vi "getPhysicalChannels.vi"(8 "error in (no error)":errorcluster, 11 "DeviceData in":refnum<class "DeviceData.lvclass">) -> (0 "error out":errorcluster, 2 "physicalChannels":string, 3 "DeviceData out":refnum<class "DeviceData.lvclass">)   [LabVIEW 2009, in "DataMappers.lvlib" / "DeviceData.lvclass"]
uses:
  DeviceData.lvclass
  Scripting/ScriptingEvent/ScriptEventList/ScriptEventList.lvclass
  DeviceData.lvclass/DeviceData.ctl
  DatabaseHelpers/Database Objects/device/device.lvclass
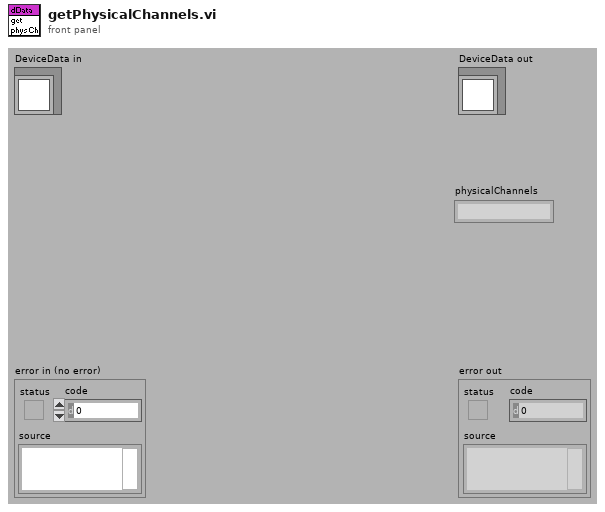
[diagram p1: front panel]
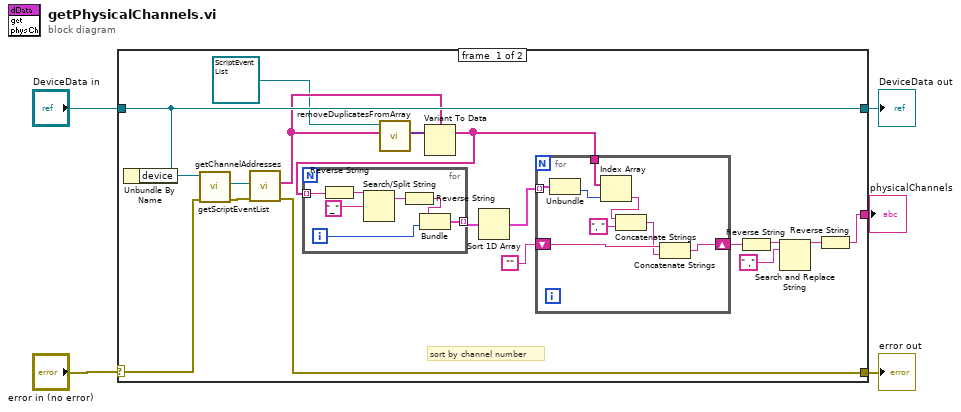
[diagram p0: block diagram]
diagram:
  n1 = case shown="No Error" "error in (no error)" {
    selector: "error in (no error)" -> [w13 w40]
    tunnel: [w12 w40] -> w4
    tunnel: [w23 w39] -> w2
    tunnel: "DeviceData in" -> [w23 w39]
    tunnel: [w14 _] -> w1
    frame #0 {
      # "sort by channel number"
      n2 = Unbundle By Name(w23) -> ("device"=w22:refnum<class "device.lvclass">)
      n3 = call "getScriptEventList.vi"("error in (no error)"=w13, "device.lvclass in"=w22) -> ("error out"=w20:errorcluster, "ScriptEventList"=w21:refnum<class "ScriptEventList.lvclass">)  [unwired: 7 in, 1 out]
      n4 = call "getChannelAddresses.vi"("error in (no error)"=w20, "ScriptEventList in"=w21) -> ("error out"=w12:errorcluster, "ChannelAddresses"=w8:string[])  [unwired: 7 in, 1 out]
      n5 = call "removeDuplicatesFromArray.vi"("Array"=w8, "ScriptEventList in"=refnum<class "ScriptEventList.lvclass"> refnum) -> ("Array out"=w9:variant[])  [unwired: 7 in, 2 out]
      n6 = Variant To Data(Variant=w9, type=w8) -> (data=w6:string[])  [unwired: 1 in, 1 out]
      n7 = for {
        tunnel: w6 -> [w30] mode=indexing
        tunnel: [w25] -> w11 mode=indexing
        i -> [w26]
        n8 = Reverse String(1:w30) -> (0:w29:string)
        n9 = Search/Split String(string=w29, search string/char (-)="_") -> (substring before match=w28:string)  [unwired: 1 in, 2 out]
        n10 = Reverse String(1:w28) -> (0:w27:string)
        n11 = Bundle(w27, w26) -> (w25:cluster{string, i32})  [unwired: 1 in]
      }
      n12 = Sort 1D Array(array=w11) -> (sorted array=w10:cluster{string, i32}[])
      n13 = for {
        shift-right: [w35] -> w18
        shift-left: "" -> [w37]
        tunnel: w10 -> [w34] mode=indexing
        tunnel: w6 -> [w32]
        n14 = Unbundle(w34) -> (w33:i32)  [unwired: 1 out]
        n15 = Index Array(array=w32, index=w33) -> (element=w31:string)
        n16 = Concatenate Strings(w31, ", ") -> (w36:string)
        n17 = Concatenate Strings(w37, w36) -> (w35:string)
      }
      n18 = Reverse String(1:w18) -> (0:w17:string)
      n19 = Search and Replace String(input string=w17, search string=" ,") -> (result string=w15:string)  [unwired: 6 in, 3 out]
      n20 = Reverse String(1:w15) -> (0:w14:string)
    }
    frame #1 {
    }
  }
  "error out" <- w4
  "DeviceData out" <- w2
  "physicalChannels" <- w1
